vi "list - get closest string.vi"(10 "number":i32, 11 "string Array":string[](array[string])) -> (0 "closest string":string, 1 "closest index":i32, 2 "closest value":i32)   [LabVIEW 2012]
uses:
  <vilib>/regexp/Match Regular Expression.xnode
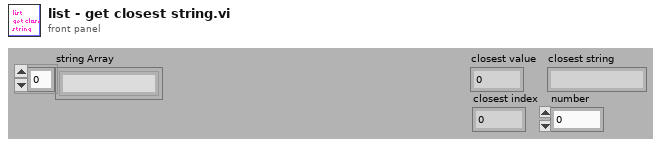
[diagram p1: front panel]
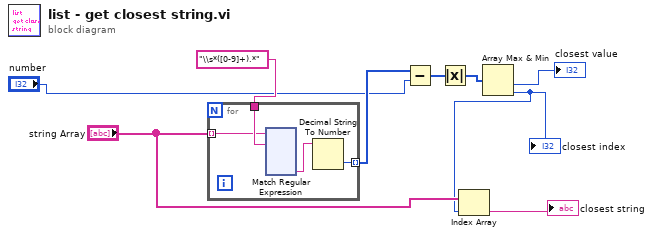
[diagram p0: block diagram]
diagram:
  n1 = for {
    tunnel: "\\s*([0-9]+).*" ("regular expression") -> [w13]
    tunnel: "string Array" -> [w12] mode=indexing
    tunnel: [w10] -> w7 mode=indexing
    n2 = xnode "Match Regular Expression"("input string"=w12, "regular expression"=w13) -> ("submatch 1"=w11:string)  [unwired: 4 in, 5 out]
    n3 = Decimal String To Number(string=w11) -> (number=w10:i32)  [unwired: 2 in, 1 out]
  }
  n4 = Subtract(x=w7, y="number") -> (x-y=w8:i32[])
  n5 = Absolute Value(x=w8) -> (abs(x)=w9:i32[])
  n6 = Array Max & Min(array=w9) -> (min value=→"closest value":i32, min index (indices)=w3:i32)  [unwired: 2 out]
  "closest index" <- w3
  n7 = Index Array(array="string Array", index=w3) -> (element=→"closest string":string)
